vi "Get Map Yaml.vi"(11 "Abstract Map Yaml Msg in":refnum<class "Abstract Map Yaml Msg.lvclass">) -> (2 "Map Yaml":T1, 3 "Abstract Map Yaml Msg out":refnum<class "Abstract Map Yaml Msg.lvclass">)   [LabVIEW 2020, in "About View.lvlib" / "Abstract Map Yaml Msg.lvclass"]
uses:
  Abstract Map Yaml Msg.lvclass
  Abstract Map Yaml Msg.lvclass/Abstract Map Yaml Msg.ctl
panel:
  # "NOTICE -- YOU MUST LEAVE THIS NOTICE IN PLACE.\n\nCopyright (c) 2017, LIANG LIU Shawn.Liu.cn@gmail.com\nAll rights reserved.\n\nRedistribution and use in source and binary forms, with or without modification, are permitted provided that the following conditions are met:\n-Redistributions of source code must retain the above copyright notice, this list of conditions and the following disclaimer.\n-Redistributions in binary form must reproduce the above copyright notice, this list of conditions and the following disclaimer in the documentation and/or other materials provided with the distribution.\n-Neither the name of the eLp nor the names of its contributors may be used to endorse or promote products derived from this software without specific prior written permission.\n\nTHIS SOFTWARE IS PROVIDED BY THE COPYRIGHT HOLDERS AND CONTRIBUTORS \"AS IS\" AND ANY EXPRESS OR IMPLIED WARRANTIES, INCLUDING, BUT NOT LIMITED TO, THE IMPLIED WARRANTIES OF MERCHANTABILITY AND FITNESS FOR A PARTICULAR PURPOSE ARE DISCLAIMED. IN NO EVENT SHALL THE COPYRIGHT HOLDER OR CONTRIBUTORS BE LIABLE FOR ANY DIRECT, INDIRECT, INCIDENTAL, SPECIAL, EXEMPLARY, OR CONSEQUENTIAL DAMAGES (INCLUDING, BUT NOT LIMITED TO, PROCUREMENT OF SUBSTITUTE GOODS OR SERVICES; LOSS OF USE, DATA, OR PROFITS; OR BUSINESS INTERRUPTION) HOWEVER CAUSED AND ON ANY THEORY OF LIABILITY, WHETHER IN CONTRACT, STRICT LIABILITY, OR TORT (INCLUDING NEGLIGENCE OR OTHERWISE) ARISING IN ANY WAY OUT OF THE USE OF THIS SOFTWARE, EVEN IF ADVISED OF THE POSSIBILITY OF SUCH DAMAGE."
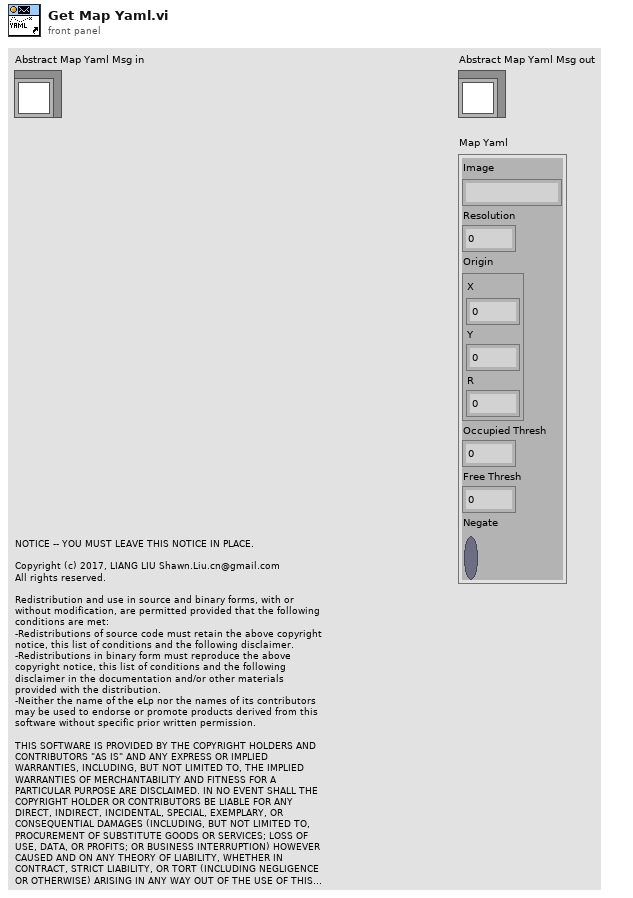
[diagram p1: front panel]
types:
  T1 = cluster{"Image":string, "Resolution":dbl, "Origin":cluster{"X":dbl, "Y":dbl, "R":dbl}, "Occupied Thresh":dbl, "Free Thresh":dbl, "Negate":bool}
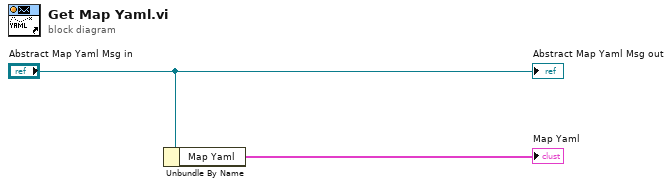
[diagram p0: block diagram]
diagram:
  n1 = Unbundle By Name("Abstract Map Yaml Msg in") -> ("Map Yaml"=→"Map Yaml":T1)
  "Abstract Map Yaml Msg out" <- "Abstract Map Yaml Msg in"
